vi "SPIM control.vi"() -> ()   [LabVIEW 2012]
uses:
  Scanning Setting.vi
panel:
  out "Peizo Voltage":dbl
  out "Peizo Location":dbl
  out "Z-Offset":dbl
  out "Scan Signal 2":cluster{"Y":dbl[], "Y":dbl[]}[](graph)
  in  "Capture":bool
  in  "DCIMG Path":path=path "H:/DATA/SET2"
  out "Frames Recorded":i32
  in  "Frames":i32=100
  out "Camera":bool=TRUE
  in  "stop":bool
  out "Image":u16[][](graph)
  in  "Snap Shut":bool
  out "Trigger":dynamicdata(graph)=[{"t0"=timestamp(16448.7 s since 1904-01-01), "dt"=1e-05, "Y"=array[10000 elements], "attributes"=variant("NI_ChannelName"=variant(string "Triangle (Collected)"), "NI_ExpIsRelativeTime"=variant(bool TRUE), "NI_ExpStartTimeStamp"=variant(timestamp timestamp(3461934223.089551 s since 1904-01-01)), "NI_ExpTimeStamp"=variant(timestamp timestamp(3461934223.089551 s since 1904-01-01)), "NI_ExpXDimension"=variant(string "t"), "NI_OriginalChannelName"=variant(string "Triangle"))}, {"t0"=timestamp(16448.7 s since 1904-01-01), "dt"=1e-05, "Y"=array[10000 elements], "attributes"=variant("NI_ChannelName"=variant(string "Square (Collected)"), "NI_ExpIsRelativeTime"=variant(bool TRUE), "NI_ExpStartTimeStamp"=variant(timestamp timestamp(3461934223.089551 s since 1904-01-01)), "NI_ExpTimeStamp"=variant(timestamp timestamp(3461934223.089551 s since 1904-01-01)), "NI_ExpXDimension"=variant(string "t"), "NI_OriginalChannelName"=variant(string "Square"))}, {"t0"=timestamp(16448.7 s since 1904-01-01), "dt"=1e-05, "Y"=array[10000 elements], "attributes"=variant("NI_ChannelName"=variant(string "Square (Collected)"), "NI_ExpIsRelativeTime"=variant(bool TRUE), "NI_ExpStartTimeStamp"=variant(timestamp timestamp(3461934223.0885506 s since 1904-01-01)), "NI_ExpTimeStamp"=variant(timestamp timestamp(3461934223.0885506 s since 1904-01-01)), "NI_ExpXDimension"=variant(string "t"), "NI_OriginalChannelName"=variant(string "Square"))}]
  out "Scan Signal":cluster{"Y":dbl[], "Y":dbl[]}[](graph)
  out "Error Out":errorcluster={"status"=TRUE, "code"=-200561, "source"="SPIM control.vi:Instance:14:1<append>\n<B>Data: </B>-10.007205\n<B>Specified Range Minimum: </B>-10.0\n<B>Specified Range Maximum: </B> 10.0\n\n<B>Task Name: </B>_unnamedTask<30>"}
  in  "Scanner":bool
  in  "Setting":bool
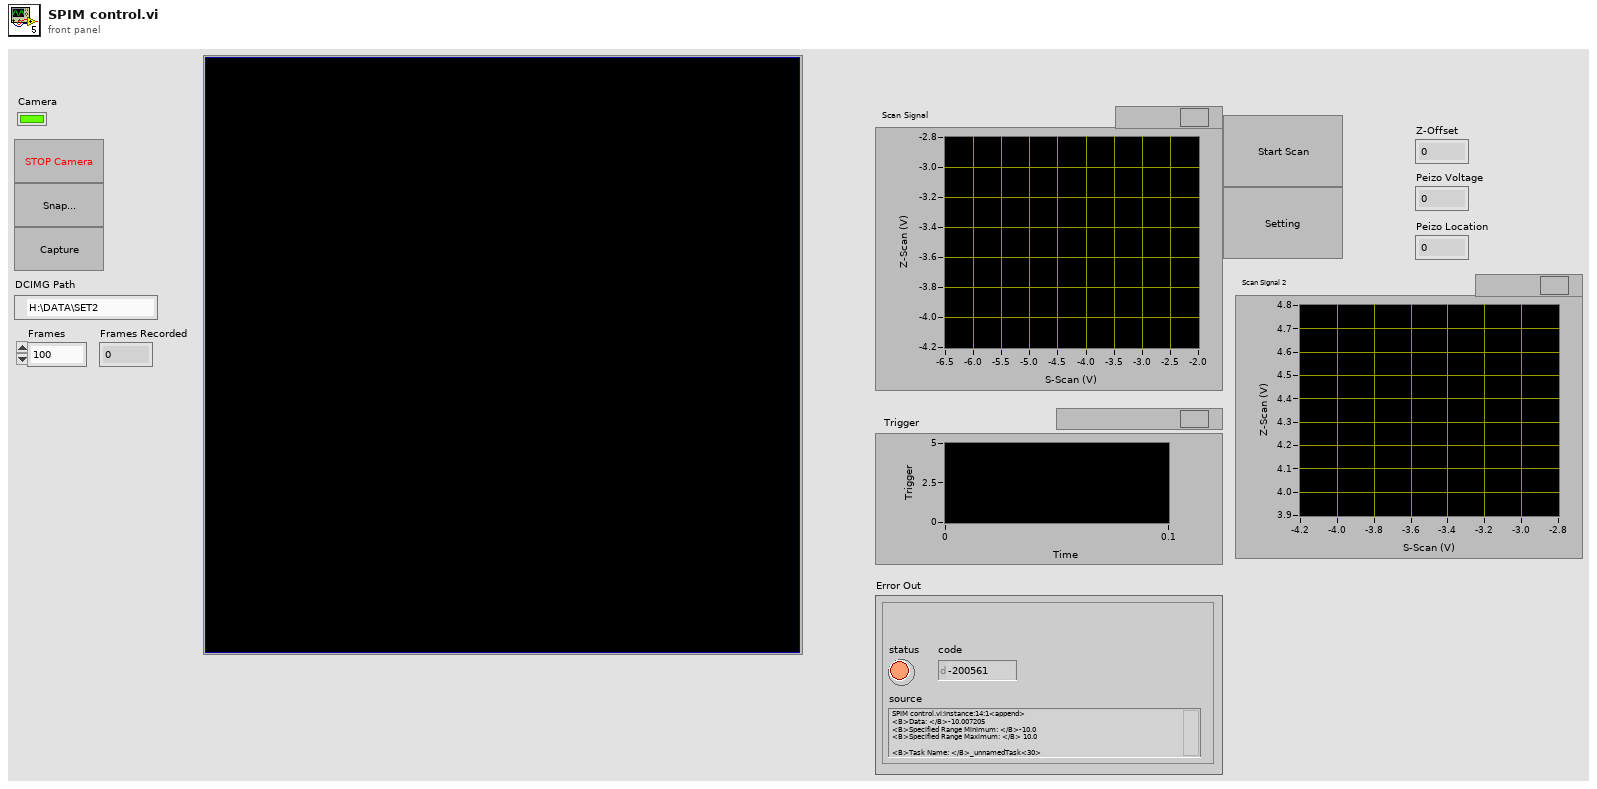
[diagram p1: front panel]
types:
  T1 = enum8{"Enabled", "Disabled", "Disabled and Grayed Out"}
  T2 = cluster{"width":u32, "height":u32, "datatype":u32}
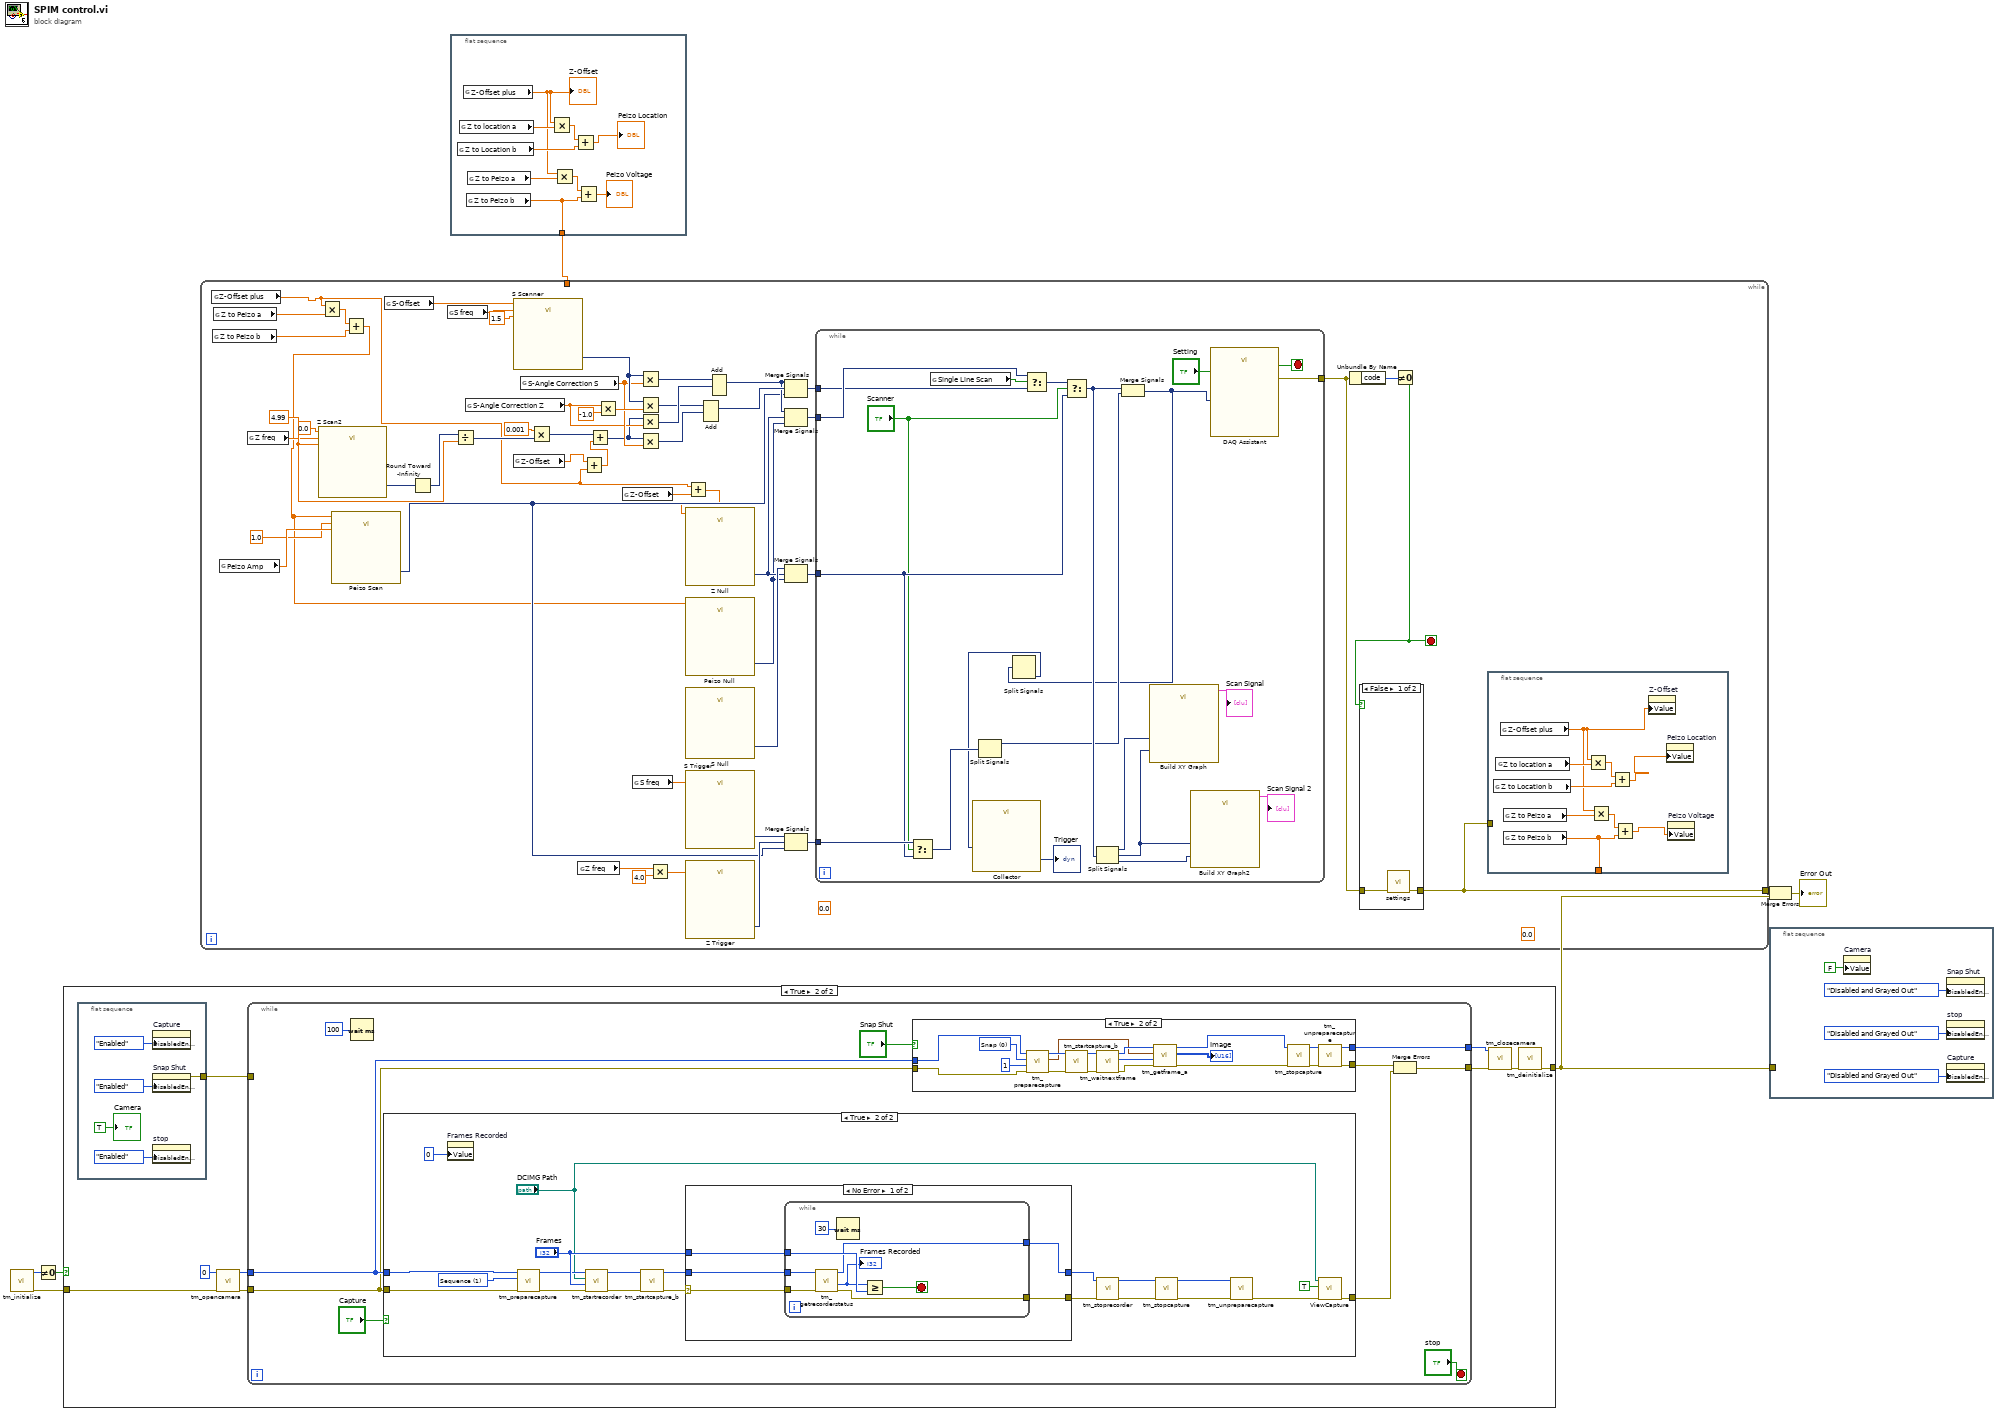
[diagram p0: block diagram]
diagram:
  n1 = call <userlib>:"tm_initialize.vi"() -> ("error out"=w4:errorcluster, "Number Of Cameras"=w5:u32)  [unwired: 10 in]
  n2 = Not Equal To 0?(x=w5) -> (x != 0?=w3:bool)
  n3 = case shown="True" w3 {
    tunnel: w4 -> [w8 w17]
    tunnel: [w8 w14] -> w2
    frame False {
    }
    frame True {
      n4 = flat-sequence {
        tunnel: [w18] -> w9
        frame #0 {
          n5 = property on="Capture" class="Bool"("DisabledEnum"=T1."Enabled" ("Disabled")) -> ()  [unwired: 2 in, 2 out]
          n6 = property on="Snap Shut" class="Bool"("DisabledEnum"=T1."Enabled" ("Disabled")) -> (error out=w18:errorcluster)  [unwired: 2 in, 1 out]
          n7 = property on="stop" class="Bool"("DisabledEnum"=T1."Enabled" ("Disabled")) -> ()  [unwired: 2 in, 2 out]
          "Camera" <- TRUE ("Camera")
        }
      }
      n8 = call <userlib>:"tm_opencamera.vi"("error in (no error)"=w17, "Camera Index"=u32 0) -> ("error out"=w10:errorcluster, "Handle out"=w11:u32)  [unwired: 8 in]
      n9 = while {
        tunnel: [w24] -> w13
        tunnel: [w32] -> w12
        tunnel: w11 -> [w28]
        tunnel: w10 -> [w27]
        tunnel: w9 -> [_]
        stop <- "stop" stop-if-true
        n10 = Wait (ms)(milliseconds to wait=u32 100) -> ()  [unwired: 1 out]
        n11 = case shown="True" "Capture" {
          tunnel: w28 -> [_ w40]
          tunnel: w27 -> [w33 w39]
          tunnel: [w33 w36] -> w26
          frame False {
          }
          frame True {
            w41 = 1 items=["Snap", "Sequence"] ("Capture mode")
            n12 = property on="Frames Recorded" class="DigNum (strict)"("Value"=0 ("Frames Recorded")) -> ()  [unwired: 2 in, 2 out]
            n13 = call <userlib>:"tm_preparecapture.vi"("error in (no error)"=w39, "Capture mode"=w41, "Handle in"=w40) -> ("error out"=w42:errorcluster, "Handle out"=w43:u32)  [unwired: 5 in, 2 out]
            n14 = call <userlib>:"tm_startrecorder.vi"("error in (no error)"=w42, "frames"="Frames", "File"="DCIMG Path", "Handle in"=w43) -> ("error out"=w44:errorcluster, "Handle out"=w45:u32)  [unwired: 6 in]
            n15 = call <userlib>:"tm_startcapture_b.vi"("error in (no error)"=w44, "Handle in"=w45) -> ("error out"=w46:errorcluster, "Handle out"=w47:u32)  [unwired: 8 in]
            n16 = case shown="No Error" w46 {
              selector: w46 -> [w59 w68]
              tunnel: w47 -> [w58 w69]
              tunnel: [w56 w69] -> w54
              tunnel: [w57 w68] -> w53
              tunnel: "Frames" -> [w55 _]
              frame No Error {
                n17 = while {
                  tunnel: w59 -> [w65]
                  tunnel: w58 -> [w64]
                  tunnel: [w63] -> w57
                  tunnel: [w66] -> w56
                  tunnel: w55 -> [w67]
                  stop <- w61 stop-if-true
                  n18 = call <userlib>:"tm_getrecorderstatus.vi"("error in (no error)"=w65, "Handle"=w64) -> ("error out"=w63:errorcluster, "Count"=w62:i32, "Handle"=w66:u32)  [unwired: 6 in, 1 out]
                  "Frames Recorded" <- w62
                  n19 = Wait (ms)(milliseconds to wait=u32 30) -> ()  [unwired: 1 out]
                  n20 = Greater Or Equal?(x=w62, y=w67) -> (x >= y?=w61:bool)
                }
              }
              frame Error {
              }
            }
            n21 = call <userlib>:"tm_stoprecorder.vi"("error in (no error)"=w53, "Handle in"=w54) -> ("error out"=w52:errorcluster, "Handle out"=w51:u32)  [unwired: 8 in]
            n22 = call <userlib>:"tm_stopcapture.vi"("error in (no error)"=w52, "Handle in"=w51) -> ("error out"=w49:errorcluster, "Handle out"=w50:u32)  [unwired: 8 in]
            n23 = call <userlib>:"tm_unpreparecapture.vi"("error in (no error)"=w49, "Handle in"=w50) -> ("error out"=w37:errorcluster)  [unwired: 8 in, 1 out]
            n24 = call "ViewCapture.vi"("error in (no error)"=w37, "Open"=TRUE, "DCIMG Path"="DCIMG Path") -> ("error out"=w36:errorcluster)  [unwired: 8 in]
          }
        }
        n25 = case shown="True" "Snap Shut" {
          tunnel: [w71 w90] -> w25
          tunnel: [w70 w89] -> w32
          tunnel: w28 -> [w70 w83]
          tunnel: w27 -> [w71 w82]
          frame False {
          }
          frame True {
            w86 = 0 items=["Snap", "Sequence"] ("Capture mode")
            n26 = call <userlib>:"tm_preparecapture.vi"("error in (no error)"=w82, "Frames"=1, "Capture mode"=w86, "Handle in"=w83) -> ("error out"=w84:errorcluster, "Buffer"=w75:T2, "Handle out"=w85:u32)  [unwired: 4 in, 1 out]
            n27 = call <userlib>:"tm_startcapture_b.vi"("error in (no error)"=w84, "Handle in"=w85) -> ("error out"=w79:errorcluster, "Handle out"=w78:u32)  [unwired: 8 in]
            n28 = call <userlib>:"tm_waitnextframe.vi"("error in (no error)"=w79, "Handle in"=w78) -> ("error out"=w77:errorcluster, "Frame Index"=w74:i32, "Handle out"=w76:u32)  [unwired: 6 in, 1 out]
            n29 = call <userlib>:"tm_getframe_a.vi"("error in (no error)"=w77, "Frame Index"=w74, "Buffer"=w75, "Handle in"=w76) -> ("error out"=w72:errorcluster, "Data 16"=→"Image":u16[][], "Handle out"=w73:u32)  [unwired: 3 in, 2 out]
            n30 = call <userlib>:"tm_stopcapture.vi"("error in (no error)"=w72, "Handle in"=w73) -> ("error out"=w87:errorcluster, "Handle out"=w88:u32)  [unwired: 8 in]
            n31 = call <userlib>:"tm_unpreparecapture.vi"("error in (no error)"=w87, "Handle in"=w88) -> ("error out"=w90:errorcluster, "Handle out"=w89:u32)  [unwired: 8 in]
          }
        }
        n32 = Merge Errors(w25, w26) -> (w24:errorcluster)
      }
      n33 = call <userlib>:"tm_closecamera.vi"("error in (no error)"=w13, "Handle in"=w12) -> ("error out"=w15:errorcluster)  [unwired: 9 in]
      n34 = call <userlib>:"tm_deinitialize.vi"("error in (no error)"=w15) -> ("error out"=w14:errorcluster)  [unwired: 10 in]
    }
  }
  n35 = while {
    tunnel: [w96] -> w7
    tunnel: w1 -> [_]
    stop <- w113 stop-if-true
    w111 = 4.99 ("Amplitude")
    (unwired) 0.0 ("Offset")
    (unwired) 0.0 ("Offset")
    n36 = global read "Scanning Setting.vi" "Z-Offset plus"() -> (w91:dbl)
    n37 = global read "Scanning Setting.vi" "Z to Peizo b"() -> (w93:dbl)
    n38 = global read "Scanning Setting.vi" "Z to Peizo a"() -> (w94:dbl)
    n39 = global read "Scanning Setting.vi" "Peizo Amp"() -> (w102:dbl)
    n40 = global read "Scanning Setting.vi" "Z freq"() -> (w104:dbl)
    n41 = call "Z Scan2"("Offset"=0.0, "Frequency"=w104, "Amplitude"=w111) -> ("Triangle"=w108:dynamicdata)  [unwired: 11 in, 1 out]
    n42 = Multiply(x=w91, y=w94) -> (x*y=w95:dbl)
    n43 = Add(x=w95, y=w93) -> (x+y=w92:dbl)
    n44 = call "Peizo Scan"("Offset"=w92, "Frequency"=1.0, "Amplitude"=w102) -> ("Sine"=w103:dynamicdata)  [unwired: 11 in, 1 out]
    n45 = global read "Scanning Setting.vi" "S-Offset"() -> (w129:dbl)
    n46 = Round Toward -Infinity(1:w108) -> (0:w109:dynamicdata)
    n47 = global read "Scanning Setting.vi" "S freq"() -> (w130:dbl)
    n48 = Divide(x=w109, y=w111) -> (x/y=w112:dynamicdata)
    n49 = global read "Scanning Setting.vi" "S-Angle Correction Z"() -> (w127:dbl)
    n50 = call "S Scanner"("Offset"=w129, "Frequency"=w130, "Amplitude"=1.5) -> ("Triangle"=w134:dynamicdata)  [unwired: 11 in, 1 out]
    n51 = global read "Scanning Setting.vi" "Z-Offset"() -> (w100:dbl)
    n52 = global read "Scanning Setting.vi" "S-Angle Correction S"() -> (w128:dbl)
    n53 = Multiply(x=0.001, y=w112) -> (x*y=w107:dynamicdata)
    n54 = global read "Scanning Setting.vi" "Z freq"() -> (w117:dbl)
    n55 = Add(x=w100, y=w91) -> (x+y=w99:dbl)
    n56 = Add(x=w107, y=w99) -> (x+y=w106:dynamicdata)
    n57 = Multiply(x=w127, y=-1.0) -> (x*y=w133:dbl)
    n58 = global read "Scanning Setting.vi" "Z-Offset"() -> (w98:dbl)
    n59 = global read "Scanning Setting.vi" "S freq"() -> (w123:dbl)
    n60 = Multiply(x=w134, y=w128) -> (x*y=w137:dynamicdata)
    n61 = Multiply(x=w134, y=w133) -> (x*y=w135:dynamicdata)
    n62 = Multiply(x=w106, y=w127) -> (x*y=w138:dynamicdata)
    n63 = Multiply(x=w106, y=w128) -> (x*y=w136:dynamicdata)
    n64 = Multiply(x=w117, y=4.0) -> (x*y=w118:dbl)
    n65 = call "Peizo Null"("Offset"=w92) -> ("Square"=w105:dynamicdata)  [unwired: 13 in, 1 out]
    n66 = call "S Null"() -> ("Triangle"=w142:dynamicdata)  [unwired: 14 in, 1 out]
    n67 = call "S Trigger"("Frequency"=w123) -> ("Square"=w122:dynamicdata)  [unwired: 13 in, 1 out]
    n68 = call "Z Trigger"("Frequency"=w118) -> ("Square"=w121:dynamicdata)  [unwired: 13 in, 1 out]
    n69 = Add(x=w91, y=w98) -> (x+y=w97:dbl)
    n70 = call "Z Null"("Offset"=w97) -> ("Square"=w126:dynamicdata)  [unwired: 13 in, 1 out]
    n71 = Add(1:w136, 2:w135) -> (0:w131:dynamicdata)  [unwired: 1 in, 1 out]
    n72 = Add(1:w138, 2:w137) -> (0:w125:dynamicdata)  [unwired: 1 in, 1 out]
    n73 = Merge Signals(w125, w131, w103) -> (w141:dynamicdata)
    n74 = Merge Signals(w125, w126, w105) -> (w124:dynamicdata)
    n75 = Merge Signals(w142, w126, w105) -> (w140:dynamicdata)
    n76 = Merge Signals(w122, w121, w103) -> (w120:dynamicdata)
    n77 = while {
      tunnel: w141 -> [w169]
      tunnel: w140 -> [w164]
      tunnel: [w173] -> w115
      tunnel: w124 -> [w171]
      tunnel: w120 -> [w165]
      stop <- w175 stop-if-true
      n78 = Select(t=w165, s="Scanner", f=w164) -> (s? t:f=w157:dynamicdata)
      n79 = global read "Scanning Setting.vi" "Single Line Scan"() -> (w170:bool)
      n80 = Split Signals(w157) -> (w158:dynamicdata)  [unwired: 3 in, 2 out]
      n81 = Select(t=w171, s=w170, f=w169) -> (s? t:f=w168:dynamicdata)
      n82 = Select(t=w168, s="Scanner", f=w164) -> (s? t:f=w167:dynamicdata)
      n83 = Split Signals(w167) -> (w160:dynamicdata, w161:dynamicdata, w159:dynamicdata)  [unwired: 3 in]
      n84 = Merge Signals(w167, w158) -> (w156:dynamicdata)
      n85 = Split Signals(w156) -> (w155:dynamicdata)  [unwired: 4 in, 3 out]
      n86 = call "Collector"("Signals"=w155) -> ("Collected Signals"=→"Trigger":dynamicdata)  [unwired: 9 in, 1 out]
      n87 = call "Build XY Graph"("Y Input"=w161, "X Input"=w160) -> ("XY Graph"=→"Scan Signal":cluster{"Y":dbl[], "Y":dbl[]}[])  [unwired: 3 in, 6 out]
      n88 = call "Build XY Graph2"("Y Input"=w159, "X Input"=w161) -> ("XY Graph"=→"Scan Signal 2":cluster{"Y":dbl[], "Y":dbl[]}[])  [unwired: 3 in, 6 out]
      n89 = call "DAQ Assistant"("data"=w156, "stop (F)"="Setting") -> ("stopped"=w175:bool, "error out"=w173:errorcluster)  [unwired: 15 in, 1 out]
    }
    n90 = Unbundle By Name(w115) -> ("code"=w114:i32)
    n91 = Not Equal To 0?(x=w114) -> (x != 0?=w113:bool)
    n92 = case shown="False" w113 {
      tunnel: [w152 w154] -> w96
      tunnel: w115 -> [w153 w154]
      frame False {
        n93 = call "settings.vi"("Error In"=w153) -> ("Error Out"=w152:errorcluster)  [unwired: 10 in]
      }
      frame True {
      }
    }
    n94 = flat-sequence {
      tunnel: [w146] -> _
      tunnel: w96 -> [_]
      frame #0 {
        n95 = global read "Scanning Setting.vi" "Z to Location b"() -> (w149:dbl)
        n96 = global read "Scanning Setting.vi" "Z to location a"() -> (w151:dbl)
        n97 = global read "Scanning Setting.vi" "Z-Offset plus"() -> (w145:dbl)
        n98 = global read "Scanning Setting.vi" "Z to Peizo b"() -> (w146:dbl)
        n99 = global read "Scanning Setting.vi" "Z to Peizo a"() -> (w147:dbl)
        n100 = Multiply(x=w145, y=w151) -> (x*y=w150:dbl)
        n101 = Multiply(x=w145, y=w147) -> (x*y=w148:dbl)
        n102 = Add(x=w150, y=w149) -> (x+y=w144:dbl)
        n103 = Add(x=w148, y=w146) -> (x+y=w143:dbl)
        n104 = property on="Z-Offset" class="DigNum (strict)"("Value"=w145) -> ()  [unwired: 2 in, 2 out]
        n105 = property on="Peizo Location" class="DigNum (strict)"("Value"=w144) -> ()  [unwired: 2 in, 2 out]
        n106 = property on="Peizo Voltage" class="DigNum (strict)"("Value"=w143) -> ()  [unwired: 2 in, 2 out]
      }
    }
  }
  n107 = flat-sequence {
    tunnel: [w176] -> w1
    frame #0 {
      n108 = global read "Scanning Setting.vi" "Z to Location b"() -> (w182:dbl)
      n109 = global read "Scanning Setting.vi" "Z to location a"() -> (w184:dbl)
      n110 = global read "Scanning Setting.vi" "Z-Offset plus"() -> (w177:dbl)
      "Z-Offset" <- w177
      n111 = global read "Scanning Setting.vi" "Z to Peizo b"() -> (w176:dbl)
      n112 = global read "Scanning Setting.vi" "Z to Peizo a"() -> (w179:dbl)
      n113 = Multiply(x=w177, y=w184) -> (x*y=w183:dbl)
      n114 = Multiply(x=w177, y=w179) -> (x*y=w180:dbl)
      n115 = Add(x=w183, y=w182) -> (x+y=→"Peizo Location":dbl)
      n116 = Add(x=w180, y=w176) -> (x+y=→"Peizo Voltage":dbl)
    }
  }
  n117 = Merge Errors(w7, w2) -> (→"Error Out":errorcluster)
  n118 = flat-sequence {
    tunnel: w2 -> [_]
    frame #0 {
      n119 = property on="Camera" class="Bool (strict)"("Value"=FALSE ("Camera")) -> ()  [unwired: 2 in, 2 out]
      n120 = property on="Snap Shut" class="Bool"("DisabledEnum"=T1."Disabled and Grayed Out" ("Disabled")) -> ()  [unwired: 2 in, 2 out]
      n121 = property on="stop" class="Bool"("DisabledEnum"=T1."Disabled and Grayed Out" ("Disabled")) -> ()  [unwired: 2 in, 2 out]
      n122 = property on="Capture" class="Bool"("DisabledEnum"=T1."Disabled and Grayed Out" ("Disabled")) -> ()  [unwired: 2 in, 2 out]
    }
  }
